vi "Get Properties.vi"(0 "hCamera IN":u32, 3 "Error IN":errorcluster) -> (5 "Pixel Format OUT":dbl, 6 "hCamera OUT":u32, 7 "Gain OUT":dbl, 8 "Colors Gain OUT":dbl[](array[numeric]) format="%.2f", 9 "Shutter Time OUT (ms)":dbl, 10 "Error OUT":errorcluster)   [LabVIEW 2010]
uses:
  <vilib>/addons/PixeLINK/Low Level Functions/CAMERA_FEATURES.llb/TDPU-CameraFeatures-FeatureIds.ctl
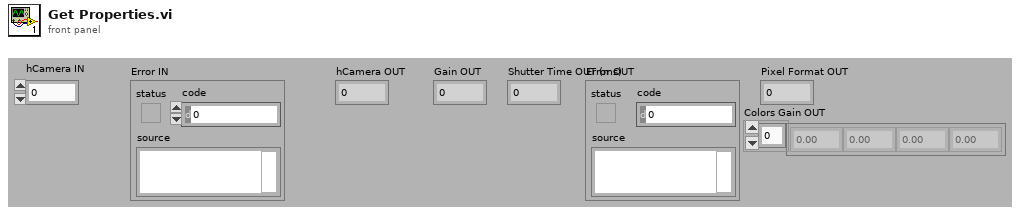
[diagram p1: front panel]
types:
  T1 = typedef "TDPU-CameraFeatures-FeatureIds.ctl" = u32
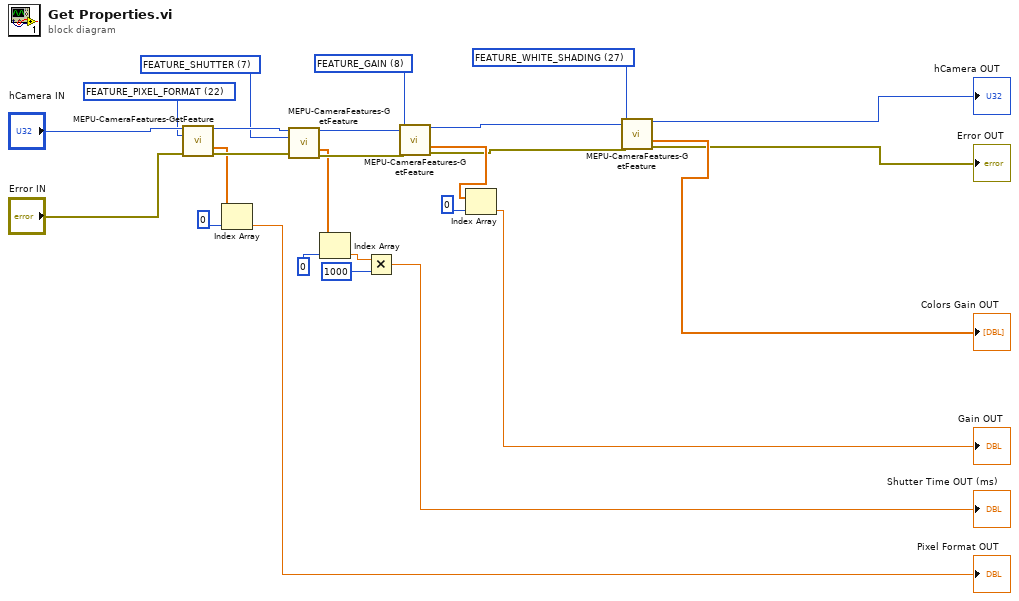
[diagram p0: block diagram]
diagram:
  w6 = T1 27 items=["FEATURE_BRIGHTNESS", "FEATURE_EXPOSURE", "FEATURE_SHARPNESS", "FEATURE_WHITE_BAL", "FEATURE_HUE", "FEATURE_SATURATION", "FEATURE_GAMMA", "FEATURE_SHUTTER", "FEATURE_GAIN", "FEATURE_IRIS", "FEATURE_FOCUS", "FEATURE_TEMPERATURE", "FEATURE_TRIGGER", "FEATURE_ZOOM", "FEATURE_PAN", "FEATURE_TILT", "FEATURE_OPT_FILTER", "FEATURE_GPIO", "FEATURE_FRAME_RATE", "FEATURE_ROI", "FEATURE_FLIP", "FEATURE_PIXEL_ADDRESSING", "FEATURE_PIXEL_FORMAT", "FEATURE_EXTENDED_SHUTTER", "FEATURE_AUTO_ROI", "FEATURE_LOOKUP_TABLE", "FEATURE_MEMORY_CHANNEL", "FEATURE_WHITE_SHADING", "FEATURE_ROTATE", "FEATURE_IMAGER_CLK_DIVISOR", "FEATURE_TRIG_WITH_CNTRLD_LIGHT", "FEATURE_MAX_PIXEL_SIZE"] ("uFeatureId IN")
  w24 = T1 8 items=["FEATURE_BRIGHTNESS", "FEATURE_EXPOSURE", "FEATURE_SHARPNESS", "FEATURE_WHITE_BAL", "FEATURE_HUE", "FEATURE_SATURATION", "FEATURE_GAMMA", "FEATURE_SHUTTER", "FEATURE_GAIN", "FEATURE_IRIS", "FEATURE_FOCUS", "FEATURE_TEMPERATURE", "FEATURE_TRIGGER", "FEATURE_ZOOM", "FEATURE_PAN", "FEATURE_TILT", "FEATURE_OPT_FILTER", "FEATURE_GPIO", "FEATURE_FRAME_RATE", "FEATURE_ROI", "FEATURE_FLIP", "FEATURE_PIXEL_ADDRESSING", "FEATURE_PIXEL_FORMAT", "FEATURE_EXTENDED_SHUTTER", "FEATURE_AUTO_ROI", "FEATURE_LOOKUP_TABLE", "FEATURE_MEMORY_CHANNEL", "FEATURE_WHITE_SHADING", "FEATURE_ROTATE", "FEATURE_IMAGER_CLK_DIVISOR", "FEATURE_TRIG_WITH_CNTRLD_LIGHT", "FEATURE_MAX_PIXEL_SIZE"] ("uFeatureId IN")
  w17 = T1 7 items=["FEATURE_BRIGHTNESS", "FEATURE_EXPOSURE", "FEATURE_SHARPNESS", "FEATURE_WHITE_BAL", "FEATURE_HUE", "FEATURE_SATURATION", "FEATURE_GAMMA", "FEATURE_SHUTTER", "FEATURE_GAIN", "FEATURE_IRIS", "FEATURE_FOCUS", "FEATURE_TEMPERATURE", "FEATURE_TRIGGER", "FEATURE_ZOOM", "FEATURE_PAN", "FEATURE_TILT", "FEATURE_OPT_FILTER", "FEATURE_GPIO", "FEATURE_FRAME_RATE", "FEATURE_ROI", "FEATURE_FLIP", "FEATURE_PIXEL_ADDRESSING", "FEATURE_PIXEL_FORMAT", "FEATURE_EXTENDED_SHUTTER", "FEATURE_AUTO_ROI", "FEATURE_LOOKUP_TABLE", "FEATURE_MEMORY_CHANNEL", "FEATURE_WHITE_SHADING", "FEATURE_ROTATE", "FEATURE_IMAGER_CLK_DIVISOR", "FEATURE_TRIG_WITH_CNTRLD_LIGHT", "FEATURE_MAX_PIXEL_SIZE"] ("uFeatureId IN")
  w8 = T1 22 items=["FEATURE_BRIGHTNESS", "FEATURE_EXPOSURE", "FEATURE_SHARPNESS", "FEATURE_WHITE_BAL", "FEATURE_HUE", "FEATURE_SATURATION", "FEATURE_GAMMA", "FEATURE_SHUTTER", "FEATURE_GAIN", "FEATURE_IRIS", "FEATURE_FOCUS", "FEATURE_TEMPERATURE", "FEATURE_TRIGGER", "FEATURE_ZOOM", "FEATURE_PAN", "FEATURE_TILT", "FEATURE_OPT_FILTER", "FEATURE_GPIO", "FEATURE_FRAME_RATE", "FEATURE_ROI", "FEATURE_FLIP", "FEATURE_PIXEL_ADDRESSING", "FEATURE_PIXEL_FORMAT", "FEATURE_EXTENDED_SHUTTER", "FEATURE_AUTO_ROI", "FEATURE_LOOKUP_TABLE", "FEATURE_MEMORY_CHANNEL", "FEATURE_WHITE_SHADING", "FEATURE_ROTATE", "FEATURE_IMAGER_CLK_DIVISOR", "FEATURE_TRIG_WITH_CNTRLD_LIGHT", "FEATURE_MAX_PIXEL_SIZE"] ("uFeatureId IN")
  n1 = call <vilib>:"MEPU-CameraFeatures-GetFeature.vi"("hCamera IN"="hCamera IN", "uFeatureId IN"=w8, "Error IN"="Error IN") -> ("hCamera OUT"=w19:u32, "pParms OUT"=w9:dbl[], "Error OUT"=w18:errorcluster)  [unwired: 8 in, 2 out]
  n2 = Index Array(array=w9, index=0) -> (element=→"Pixel Format OUT":dbl)
  n3 = call <vilib>:"MEPU-CameraFeatures-GetFeature.vi"("hCamera IN"=w19, "uFeatureId IN"=w17, "Error IN"=w18) -> ("hCamera OUT"=w23:u32, "pParms OUT"=w16:dbl[], "Error OUT"=w22:errorcluster)  [unwired: 8 in, 2 out]
  n4 = Index Array(array=w16, index=0) -> (element=w13:dbl)
  n5 = Multiply(x=w13, y=1000) -> (x*y=→"Shutter Time OUT (ms)":dbl)
  n6 = call <vilib>:"MEPU-CameraFeatures-GetFeature.vi"("hCamera IN"=w23, "uFeatureId IN"=w24, "Error IN"=w22) -> ("hCamera OUT"=w5:u32, "pParms OUT"=w26:dbl[], "Error OUT"=w4:errorcluster)  [unwired: 8 in, 2 out]
  n7 = Index Array(array=w26, index=0) -> (element=→"Gain OUT":dbl)
  n8 = call <vilib>:"MEPU-CameraFeatures-GetFeature.vi"("hCamera IN"=w5, "uFeatureId IN"=w6, "Error IN"=w4) -> ("hCamera OUT"=→"hCamera OUT":u32, "pParms OUT"=→"Colors Gain OUT":dbl[], "Error OUT"=→"Error OUT":errorcluster)  [unwired: 8 in, 2 out]
